vi "QueryServer_GetRequest_Invoke.vi"(6 "error in (no error)":errorcluster, 9 "gRPCid":T1) -> (0 "error out":errorcluster, 1 "parameter":string, 2 "command":string, 3 "gRPCid out":T1)   [LabVIEW 2019, in "labview-grpc-query-server.lvlib"]
uses:
  labview-grpc-query-server.lvlib
  VIs/grpcId.ctl
  QueryServer_InvokeRequest.ctl
  b7f627e9-e0c6-4021-9d74-0376170880ad.vi
  VIs/gprc-support.lvlib
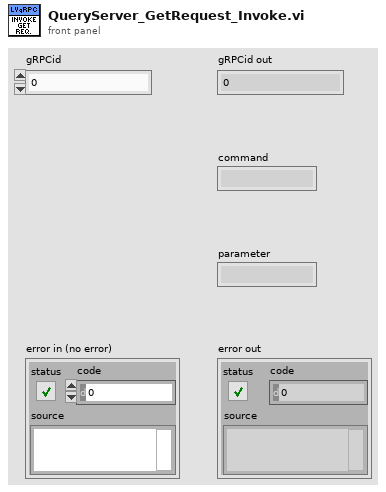
[diagram p1: front panel]
types:
  T1 = typedef "gprc-support.lvlib/grpcId.ctl" = u64
  T2 = typedef "labview-grpc-query-server.lvlib/QueryServer_InvokeRequest.ctl" = cluster{"command":string, "parameter":string}
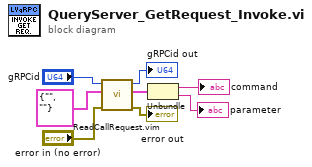
[diagram p0: block diagram]
diagram:
  n1 = call "ReadCallRequest.vim"("error in (no error)"="error in (no error)", "Data Type"=T2 {"command"="", "parameter"=""} ("InvokeRequest"), "gRPCid in"="gRPCid") -> ("error out"=→"error out":errorcluster, "Request Data"=w5:T2, "gRPCid out"=→"gRPCid out":T1)  [unwired: 6 in]
  n2 = Unbundle(w5) -> ("command"=→"command":string, "parameter"=→"parameter":string)
